vi "MSEval_main.vi"() -> ()   [LabVIEW 2015]
doc: "Main Program MSEval.\n\nAt program start the software loads the preferences and automatically\nloads available data files from the data source (folder or database)."
uses:
  Classes/AnalysisList/AnalysisList.lvclass
  MSControl/Classes/Plots/Plots.lvclass
  global_variables.vi
  Classes/AnalysisListItems/AnalysisListItems.lvclass
panel:
  in  "Recall button":bool
  in  "RunSeries Standards button":bool
  in  "export button":bool
  out "error out":errorcluster
  in  "error in (no error)":errorcluster
  in  "update button":bool
  in  "Analysis List":i32[](listbox)
  # "MS Eval"
  # "Recall Analysis"
  # "Analysis Series"
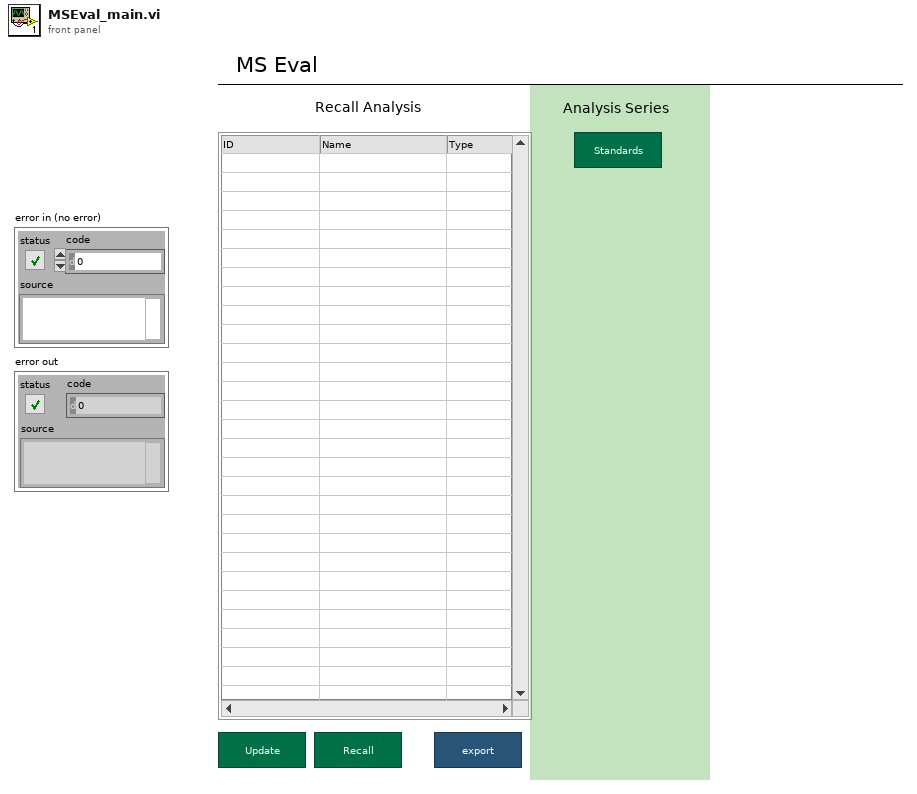
[diagram p1: front panel]
types:
  T1 = typedef "eventvkey.ctl" = enum16{"ASCII", "Enter", "Return", "Shift", "Ctrl", "Alt", "Cmd", "Opt", "Caps", "NumLock", "Clear", "Break", "Up", "Down", "Left", "Right", "Insert", "Delete", "Home", "End", "PageUp", "PageDown", "Escape", "Help", "Pause", "ScrollLock", "F1", "F2", "F3", "F4", "F5", "F6", "F7", "F8", "F9", "F10", "F11", "F12", "F13", "F14", "F15", "F16", "F17", "F18", "F19", "F20", "F21", "F22", "F23", "F24", "Play", "VolumeUp", "VolumeDown", "Mute", "Two Byte Char"}
  T2 = cluster{"Shift":bool, "Ctrl":bool, "Alt":bool, "Cmd":bool, "Opt":bool}
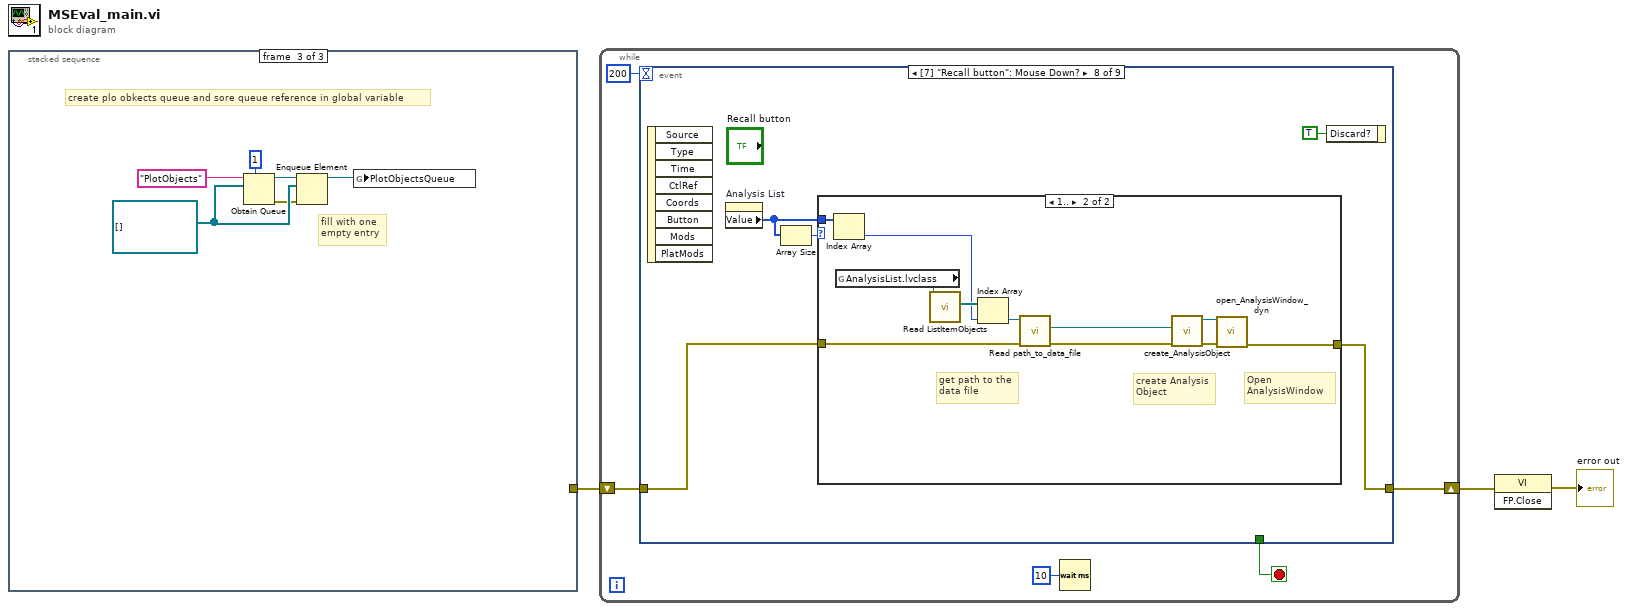
[diagram p0: block diagram]
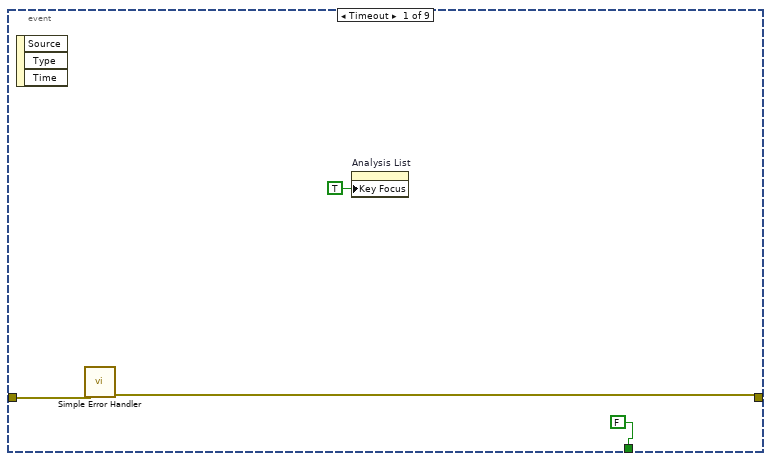
[diagram p2: hidden frame]
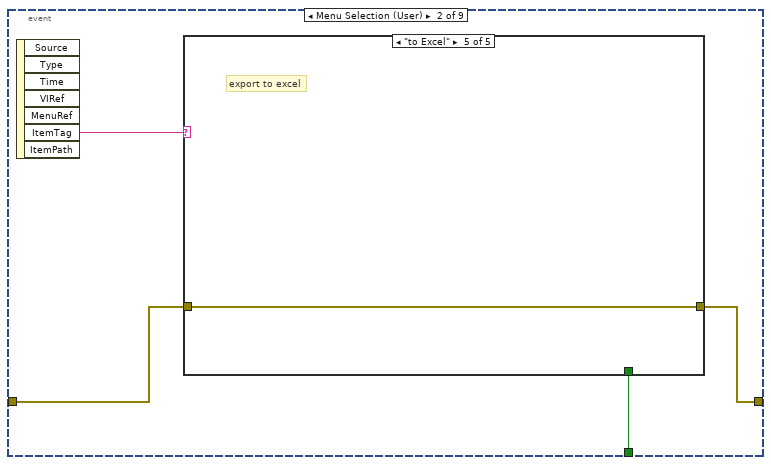
[diagram p3: hidden frame]
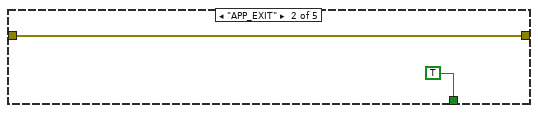
[diagram p5: hidden frame]
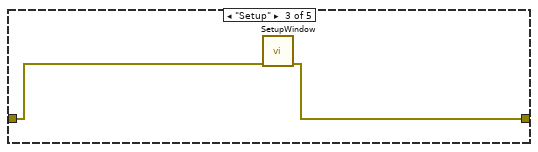
[diagram p6: hidden frame]
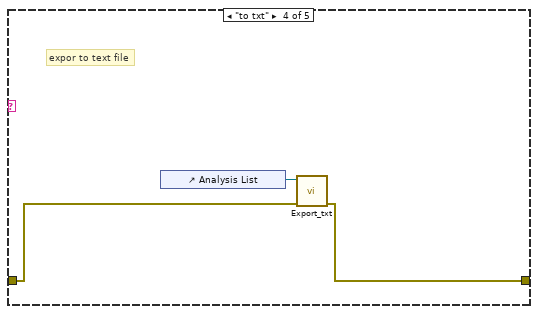
[diagram p7: hidden frame]
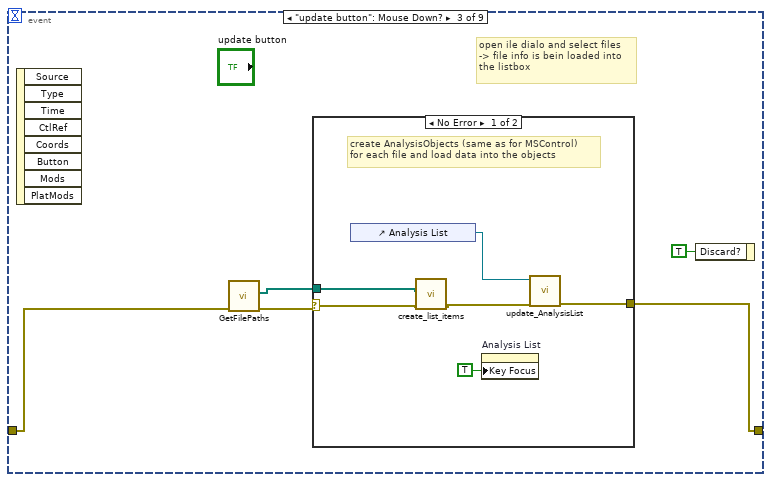
[diagram p8: hidden frame]
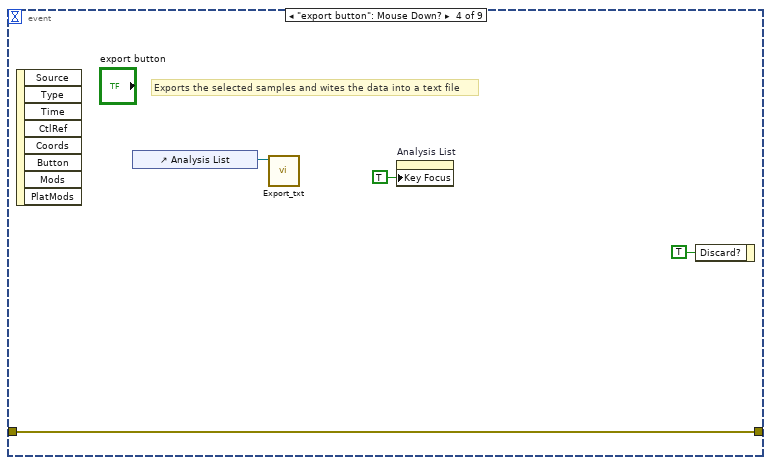
[diagram p10: hidden frame]
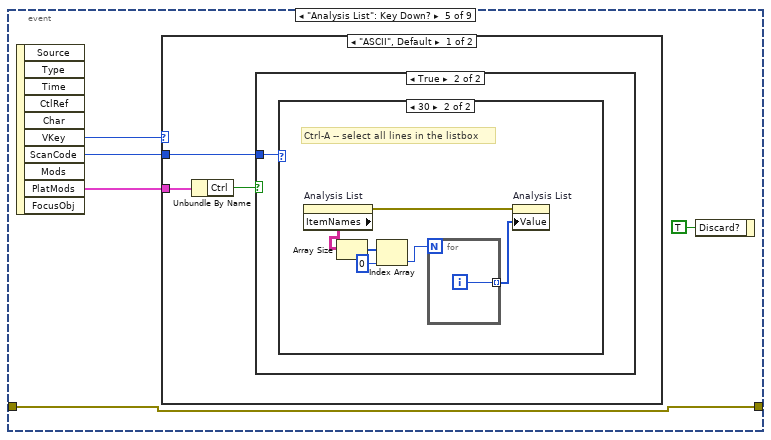
[diagram p11: hidden frame]
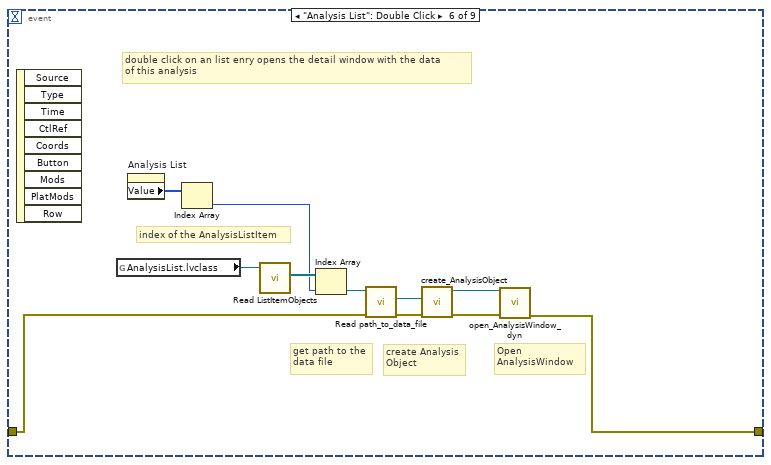
[diagram p15: hidden frame]
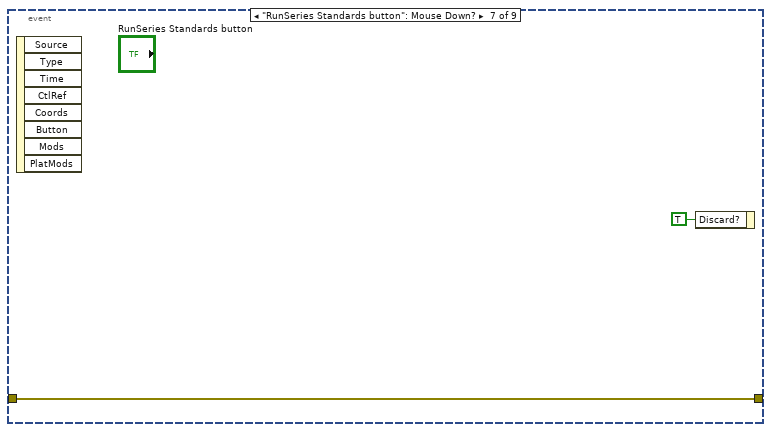
[diagram p16: hidden frame]
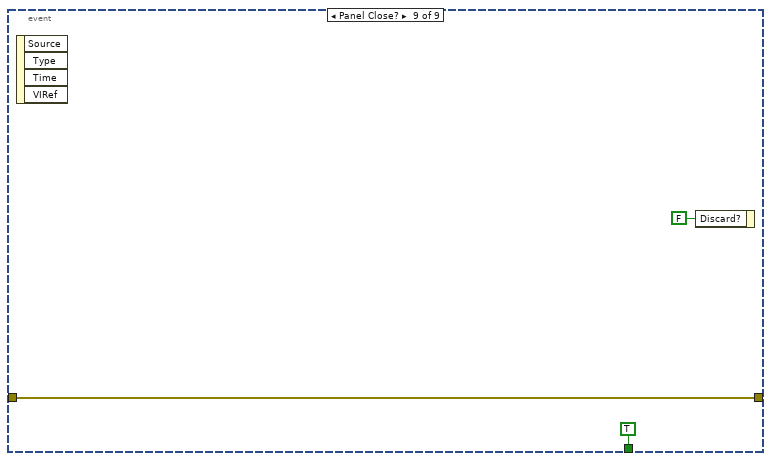
[diagram p18: hidden frame]
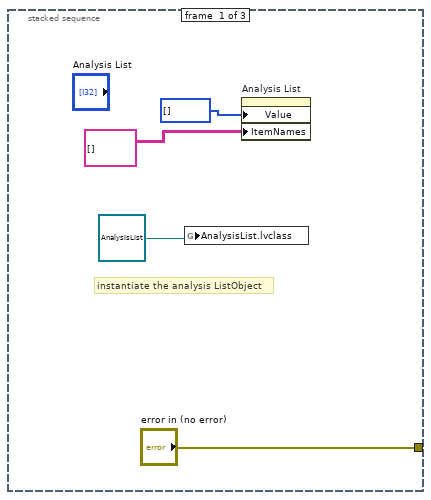
[diagram p19: hidden frame]
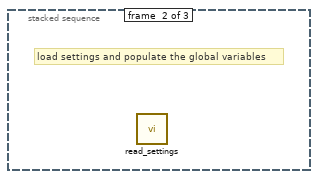
[diagram p20: hidden frame]
diagram:
  n1 = stacked-sequence {
    tunnel: ["error in (no error)" _ _] -> w3
    frame #0 {
      # "instantiate the analysis ListObject"
      n2 = global write "global_variables.vi" "AnalysisList.lvclass"(refnum<class "AnalysisList.lvclass"> refnum ("AnalysisList.lvclass")) -> ()
      n3 = property on="Analysis List" class="MCListbox (strict)"("Value"=i32[] [], "ItemNames"=string[][] []) -> ()  [unwired: 2 in, 2 out]
    }
    frame #1 {
      # "load settings and populate the global variables"
      n4 = call "read_settings.vi"() -> ()  [unwired: 11 in, 1 out]
    }
    frame #2 {
      w10 = refnum<class "Plots.lvclass">[] [] ("PlotObjArray")
      # "fill with one\nempty entry"
      # "create plo obkects queue and sore queue reference in global variable"
      n5 = Obtain Queue(max queue size (-1, unlimited)=1, name (unnamed)="PlotObjects", element data type=w10) -> (queue out=w11:refnum<queue>, error out=w9:errorcluster)  [unwired: 2 in, 1 out]
      n6 = Enqueue Element(queue=w11, element=w10, error in (no error)=w9) -> (queue out=w8:refnum<queue>)  [unwired: 1 in, 2 out]
      n7 = global write "global_variables.vi" "PlotObjectsQueue"(w8) -> ()
    }
  }
  n8 = while {
    shift-right: [w16] -> w2
    shift-left: w3 -> [w18]
    stop <- w17 stop-if-true
    n9 = event shown="[7] \"Recall button\": Mouse Down?" {
      selector: _ -> [_ _ _ _ _ _ _ _ _]
      dyn-events: _ -> [_ _ _ _ _ _ _ _ _]
      timeout: 200 -> [_ _ _ _ _ _ _ _ _]
      tunnel: w18 -> [w20 w24 w39 w48 w52 w70 w79 w84 w98]
      tunnel: [FALSE w25 _ _ _ _ _ _ TRUE] -> w17
      tunnel: [w19 w23 w36 w48 w52 w78 w79 w83 w98] -> w16
      event Timeout {
        n10 = event-data() -> ()  [unwired: 1 in, 3 out]
        n11 = call <vilib>:"Simple Error Handler.vi"("error in (no error)"=w20) -> ("error out"=w19:errorcluster)  [unwired: 4 in, 4 out]
        n12 = property on="Analysis List" class="MCListbox (strict)"("Key Focus"=TRUE) -> ()  [unwired: 2 in, 2 out]
      }
      event Menu Selection (User) {
        n13 = event-data() -> ("ItemTag"=w26:string)  [unwired: 1 in, 6 out]
        n14 = case shown="\"to Excel\"" w26 {
          tunnel: [_ TRUE _ _ _] -> w25
          tunnel: w24 -> [w27 w28 w31 w33 w35]
          tunnel: [w27 w28 w30 w32 w35] -> w23
          frame "False", Default {
          }
          frame "APP_EXIT" {
          }
          frame "Setup" {
            n15 = call "SetupWindow.vi"("error in (no error)"=w31) -> ("error out"=w30:errorcluster)  [unwired: 10 in]
          }
          frame "to txt" {
            # "expor to text file"
            n16 = control-ref of="Analysis List"() -> (w34:refnum<vi>)
            n17 = call "Export_txt.vi"("error in (no error)"=w33, "Analysis List ref"=w34) -> ("error out"=w32:errorcluster)  [unwired: 9 in]
          }
          frame "to Excel" {
            # "export to excel"
          }
        }
      }
      event "update button": Mouse Down? {
        # "open ile dialo and select files\n-> file info is bein loaded into\nthe listbox"
        n18 = event-data() -> ()  [unwired: 1 in, 8 out]
        n19 = call "GetFilePaths.vi"("error in (no error)"=w39) -> ("error out"=w38:errorcluster, "FilePaths out"=w37:path[])  [unwired: 9 in]
        n20 = case shown="No Error" w38 {
          selector: w38 -> [w42 w47]
          tunnel: w37 -> [w43 _]
          tunnel: [w44 w47] -> w36
          frame No Error {
            # "create AnalysisObjects (same as for MSControl)\nfor each file and load data into the objects"
            n21 = control-ref of="Analysis List"() -> (w46:refnum<vi>)
            n22 = call "create_list_items.vi"("error in (no error)"=w42, "FilePaths"=w43) -> ("error out"=w41:errorcluster)  [unwired: 9 in]
            n23 = property on="Analysis List" class="MCListbox (strict)"("Key Focus"=TRUE) -> ()  [unwired: 2 in, 2 out]
            n24 = call "update_AnalysisList.vi"("error in (no error)"=w41, "Analysis List ref"=w46) -> ("error out"=w44:errorcluster)  [unwired: 9 in]
          }
          frame Error {
            # "dialog is canelled"
          }
        }
        n25 = event-data("Discard?"=TRUE) -> ()  [unwired: 1 in, 1 out]
      }
      event "export button": Mouse Down? {
        # "Exports the selected samples and wites the data into a text file"
        n26 = event-data() -> ()  [unwired: 1 in, 8 out]
        n27 = control-ref of="Analysis List"() -> (w49:refnum<vi>)
        n28 = call "Export_txt.vi"("Analysis List ref"=w49) -> ()  [unwired: 10 in, 1 out]
        n29 = property on="Analysis List" class="MCListbox (strict)"("Key Focus"=TRUE) -> ()  [unwired: 2 in, 2 out]
        n30 = event-data("Discard?"=TRUE) -> ()  [unwired: 1 in, 1 out]
      }
      event "Analysis List": Key Down? {
        n31 = event-data() -> ("VKey"=w56:T1, "ScanCode"=w54:i16, "PlatMods"=w55:T2)  [unwired: 1 in, 7 out]
        n32 = case shown="\"ASCII\", Default" w56 {
          tunnel: w55 -> [w59 _]
          tunnel: w54 -> [w57 _]
          frame "ASCII", Default {
            n33 = Unbundle By Name(w59) -> ("Ctrl"=w58:bool)
            n34 = case shown="True" w58 {
              tunnel: w57 -> [_ w60]
              frame False {
              }
              frame True {
                n35 = case shown="30" w60 {
                  frame 0, Default {
                  }
                  frame 30 {
                    # "Ctrl-A -- select all lines in the listbox"
                    n36 = property on="Analysis List" class="MCListbox (strict)"() -> (error out=w61:errorcluster, "ItemNames"=w66:string[][])  [unwired: 2 in, 1 out]
                    n37 = Array Size(array=w66) -> (size(s)=w65:i32[])
                    n38 = Index Array(array=w65, index=0) -> (element=w63:i32)
                    n39 = for {
                      N: w63 -> [_]
                      tunnel: [w67] -> w62 mode=indexing
                      i -> [w67]
                    }
                    n40 = property on="Analysis List" class="MCListbox (strict)"(error in=w61, "Value"=w62) -> ()  [unwired: 1 in, 2 out]
                  }
                }
              }
            }
          }
          frame "Enter" {
          }
        }
        n41 = event-data("Discard?"=TRUE) -> ()  [unwired: 1 in, 1 out]
      }
      event "Analysis List": Double Click {
        # "Open\nAnalysisWindow"
        # "create Analysis\nObject"
        # "get path to the\ndata file"
        # "index of the AnalysisListItem"
        # "double click on an list enry opens the detail window with the data\nof this analysis"
        n42 = event-data() -> ()  [unwired: 1 in, 9 out]
        n43 = global read "global_variables.vi" "AnalysisList.lvclass"() -> (w76:refnum<class "AnalysisList.lvclass">)
        n44 = property on="Analysis List" class="MCListbox (strict)"() -> ("Value"=w77:i32[])  [unwired: 2 in, 2 out]
        n45 = Index Array(array=w77) -> (element=w74:i32)  [unwired: 1 in]
        n46 = call-dynamic "Read ListItemObjects.vi"("AnalysisList in"=w76) -> ("AnalysisObjects"=w75:refnum<class "AnalysisListItems.lvclass">[])  [unwired: 8 in, 2 out]
        n47 = Index Array(array=w75, index=w74) -> (element=w73:refnum<class "AnalysisListItems.lvclass">)
        n48 = call-dynamic "Read path_to_data_file.vi"("error in (no error)"=w70, "AnalysisListItems in"=w73) -> ("error out"=w71:errorcluster, "path_to_data_file"=w72:path)  [unwired: 7 in, 1 out]
        n49 = call "create_AnalysisObject.vi"("error in (no error)"=w71, "FilePath"=w72) -> ("error out"=w68:errorcluster, "Analysis out"=w69:refnum<class "Analysis.lvclass">)  [unwired: 8 in]
        n50 = call "open_AnalysisWindow_dyn.vi"("error in (no error)"=w68, "Analysis in"=w69) -> ("error out"=w78:errorcluster)  [unwired: 9 in]
      }
      event "RunSeries Standards button": Mouse Down? {
        n51 = event-data() -> ()  [unwired: 1 in, 8 out]
        n52 = event-data("Discard?"=TRUE) -> ()  [unwired: 1 in, 1 out]
      }
      event "Recall button": Mouse Down? {
        n53 = event-data() -> ()  [unwired: 1 in, 8 out]
        n54 = property on="Analysis List" class="MCListbox (strict)"() -> ("Value"=w81:i32[])  [unwired: 2 in, 2 out]
        n55 = Array Size(array=w81) -> (size(s)=w82:i32)
        n56 = case shown="1.." w82 {
          tunnel: w84 -> [w86 w90]
          tunnel: [w86 w89] -> w83
          tunnel: w81 -> [_ w88]
          frame 0, Default {
            # "nothin selected"
          }
          frame 1.. {
            # "Open\nAnalysisWindow"
            # "create Analysis\nObject"
            # "get path to the\ndata file"
            n57 = Index Array(array=w88) -> (element=w87:i32)  [unwired: 1 in]
            n58 = global read "global_variables.vi" "AnalysisList.lvclass"() -> (w97:refnum<class "AnalysisList.lvclass">)
            n59 = call-dynamic "Read ListItemObjects.vi"("AnalysisList in"=w97) -> ("AnalysisObjects"=w96:refnum<class "AnalysisListItems.lvclass">[])  [unwired: 8 in, 2 out]
            n60 = Index Array(array=w96, index=w87) -> (element=w95:refnum<class "AnalysisListItems.lvclass">)
            n61 = call-dynamic "Read path_to_data_file.vi"("error in (no error)"=w90, "AnalysisListItems in"=w95) -> ("error out"=w93:errorcluster, "path_to_data_file"=w94:path)  [unwired: 7 in, 1 out]
            n62 = call "create_AnalysisObject.vi"("error in (no error)"=w93, "FilePath"=w94) -> ("error out"=w91:errorcluster, "Analysis out"=w92:refnum<class "Analysis.lvclass">)  [unwired: 8 in]
            n63 = call "open_AnalysisWindow_dyn.vi"("error in (no error)"=w91, "Analysis in"=w92) -> ("error out"=w89:errorcluster)  [unwired: 9 in]
          }
        }
        n64 = event-data("Discard?"=TRUE) -> ()  [unwired: 1 in, 1 out]
      }
      event Panel Close? {
        n65 = event-data() -> ()  [unwired: 1 in, 4 out]
        n66 = event-data("Discard?"=FALSE) -> ()  [unwired: 1 in, 1 out]
      }
    }
    n67 = Wait (ms)(milliseconds to wait=u32 10) -> ()  [unwired: 1 out]
  }
  n68 = invoke class="VI" method="FP.Close"(error in=w2) -> (error out=→"error out":errorcluster)  [unwired: 2 in, 2 out]
